vi "List to 1D Array.vi"(11 "List String":string) -> (3 "1D Array":string[](array[string]))   [LabVIEW 2020]
uses:
  ccd404da-7605-4e00-af1a-43a10f3ce970.vi
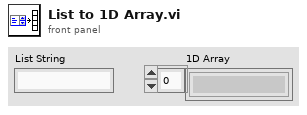
[diagram p1: front panel]
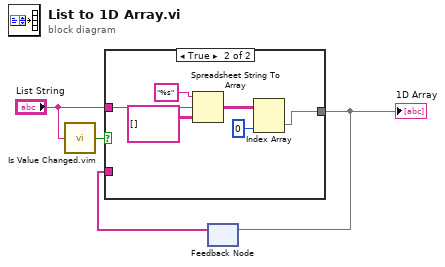
[diagram p0: block diagram]
diagram:
  n1 = call "Is Value Changed.vim"("value"="List String") -> ("changed or first call?"=w1:bool)
  n2 = feedback #1() -> (w3:string[])  [unwired: 1 in]
  n3 = case shown="True" w1 {
    tunnel: [w5 w6] -> w4
    tunnel: "List String" -> [_ w11]
    tunnel: w3 -> [w5 _]
    frame False {
    }
    frame True {
      n4 = Spreadsheet String To Array(format string="%s", spreadsheet string=w11, array type (2D Dbl)=string[][] [] ("format string")) -> (array=w8:string[][])  [unwired: 1 in]
      n5 = Index Array(array=w8, index (col)=0 ("disabled index (col)")) -> (element=w6:string[])  [unwired: 1 in]
    }
  }
  "1D Array" <- w4
  n6 = feedback-in #1(w4) -> ()
